vi "r-note.vi"(11 "Cluster":T1) -> (3 "String":string)   [LabVIEW 2019]
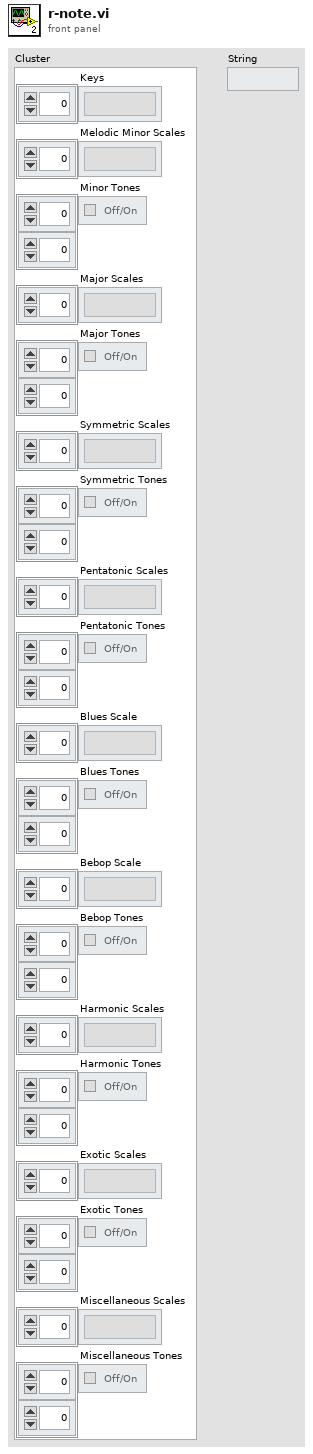
[diagram p1: front panel]
types:
  T1 = cluster{"Keys":string[], "Melodic Minor Scales":string[], "Minor Tones":bool[][], "Major Scales":string[], "Major Tones":bool[][], "Symmetric Scales":string[], "Symmetric Tones":bool[][], "Pentatonic Scales":string[], "Pentatonic Tones":bool[][], "Blues Scale":string[], "Blues Tones":bool[][], "Bebop Scale":string[], "Bebop Tones":bool[][], "Harmonic Scales":string[], "Harmonic Tones":bool[][], "Exotic Scales":string[], "Exotic Tones":bool[][], "Miscellaneous Scales":string[], "Miscellaneous Tones":bool[][]}
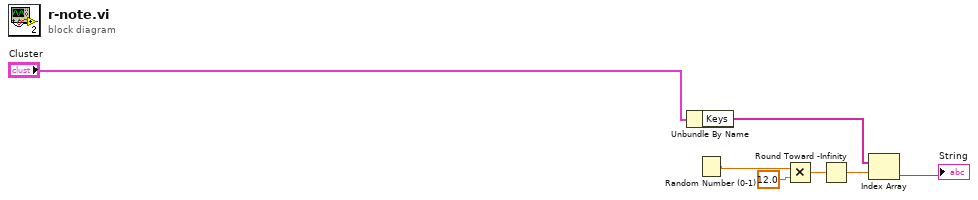
[diagram p0: block diagram]
diagram:
  n1 = Unbundle By Name("Cluster") -> ("Keys"=w5:string[])
  n2 = Random Number (0-1)() -> (number: 0 to 1=w7:dbl)
  n3 = Multiply(x=w7, y=12.0) -> (x*y=w2:dbl)
  n4 = Round Toward -Infinity(1:w2) -> (0:w1:dbl)
  n5 = Index Array(array=w5, index=w1) -> (element=→"String":string)
